vi "Choose error bar type.vi"(3 "Error_bars":T2, 4 "Error Bars":T1, 5 "Error Bar Type":T3=enum."Standard Error") -> (0 "Lower":string[](array[string]), 1 "Lower Upper":i32[](array[numeric]), 2 "Upper":string[](array[string]))   [LabVIEW 2018]
uses:
  Error bar Type.ctl
  Error_bars.ctl
  Error_bars_index.ctl
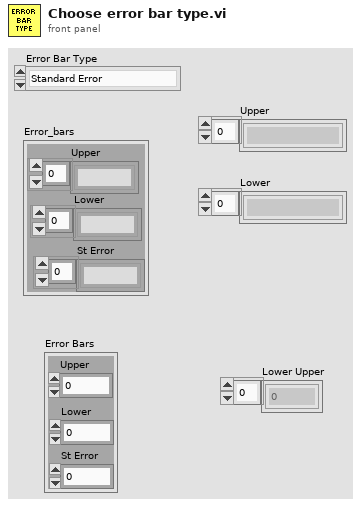
[diagram p1: front panel]
types:
  T1 = typedef "Error_bars_index.ctl" = cluster{"Upper":i32, "Lower":i32, "St Error":i32}
  T2 = typedef "Error_bars.ctl" = cluster{"Upper":string[], "Lower":string[], "St Error":string[]}
  T3 = typedef "Error bar Type.ctl" = enum16{"None", "Standard Error", "Separate upper and lower"}
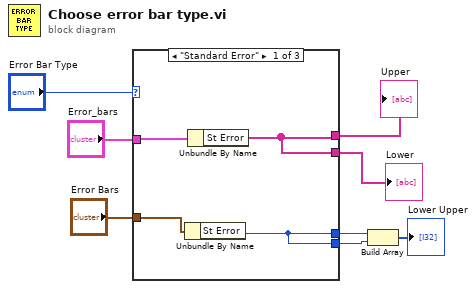
[diagram p0: block diagram]
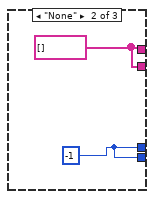
[diagram p2: hidden frame]
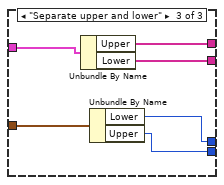
[diagram p3: hidden frame]
diagram:
  n1 = case shown="\"Standard Error\"" "Error Bar Type" {
    tunnel: "Error_bars" -> [w12 _ w20]
    tunnel: [w11 w14 w19] -> w6
    tunnel: [w11 w14 w18] -> w5
    tunnel: "Error Bars" -> [w10 _ w17]
    tunnel: [w9 w13 w16] -> w3
    tunnel: [w9 w13 w15] -> w2
    frame "Standard Error" {
      n2 = Unbundle By Name(w10) -> ("St Error"=w9:i32)
      n3 = Unbundle By Name(w12) -> ("St Error"=w11:string[])
    }
    frame "None" {
      w13 = -1 ("St Error")
      w14 = string[] [] ("Upper")
    }
    frame "Separate upper and lower" {
      n4 = Unbundle By Name(w20) -> ("Upper"=w19:string[], "Lower"=w18:string[])
      n5 = Unbundle By Name(w17) -> ("Lower"=w16:i32, "Upper"=w15:i32)
    }
  }
  "Upper" <- w6
  "Lower" <- w5
  n6 = Build Array(w3, w2) -> (→"Lower Upper":i32[])
